vi "FFT Simulation test.vi"   [LabVIEW 2014]
uses:
  <vilib>/Platform/TimedLoop/XDataNode/timing_clust.ctl
  <vilib>/Platform/TimedLoop/XDataNode/nitl_modes.ctl
  <vilib>/Platform/TimedLoop/XDataNode/wakeup.ctl
  <vilib>/rvi/Analysis/measure/FFT/simModelSupport/niFPGA FFT Streaming Sim Properties.ctl
  <vilib>/rvi/Analysis/measure/FFT/simModelSupport/niFPGA FFT Sim Stream Group Properties.ctl
  <vilib>/rvi/Analysis/measure/FFT/simModelSupport/niFPGA FFT Sim Types.ctl
  <vilib>/rvi/Analysis/measure/FFT/simModelSupport/niFpgaFFTSimArithmeticProperties.ctl
  <vilib>/rvi/Analysis/measure/FFT/simModelSupport/niFpgaFFTSimDfxp.ctl
  <vilib>/fxp/LVFixedPointQuantizationPolicyTypeDef.ctl
  <vilib>/rvi/Analysis/measure/FFT/XNode/niFpgaFFTButterflyDelays.ctl
  <vilib>/rvi/Emulation/niFpgaSctlEmulationGetInTimedLoop.vi
  <vilib>/rvi/Emulation/niFpgaEmulationReportErrorSimple.vi
  <vilib>/rvi/Emulation/niFpgaGetClockAttributes.vi
  <vilib>/rvi/Emulation/niFpgaCriticalErrorInLSC.vi
  <vilib>/rvi/Memory/Memory_Emulation/nirvimemoryFastEmulation.vi
  <vilib>/rvi/Memory/Memory_Emulation/nirvimemoryEmulation.vi
  <vilib>/rvi/Emulation/niFpgaEmulationIsFPGAContextNoSignature.vi
  <vilib>/rvi/DataTransferAndStorage/Container/Common/niFpgaContainerGetUniqueNameForEmu.vi
  <vilib>/rvi/Emulation/niFpgaProcessEmulError.vi
  <vilib>/rvi/errors/nirviReportUnexpectedCaseInternalError (U32).vi
  <vilib>/rvi/interface/RandomDataEmulation/niFpgaRandomDataHandleErrors.vi
  <vilib>/rvi/errors/niFpgaSetErrorForExecOnDevCompSimple.vi
  <vilib>/rvi/eio/common/nirviEmuReportErrorAndStop.vi
  <vilib>/rvi/FIFO/Fifo_Resource/nirvififoEmulationSetSize.vi
  <vilib>/rvi/FIFO/Fifo_Resource/nirviFifoEmulationQueueMgr.vi
  <instcachedir>/0/nirviFifoEmulationQueueMgr_E5CAEC123FF24DC58D834DCA3CDAA9B5.lvgen/nirviFifoEmulationQueueMgr_E5CAEC123FF24DC58D834DCA3CDAA9B5_010.vi
  <vilib>/rvi/FIFO/Fifo_Resource/nirvififoEmulationDetermineInputValidOut.vi
  <vilib>/rvi/FIFO/Fifo_Resource/nirvififoEmulationCreateLock.vi
  <vilib>/rvi/FIFO/Fifo_Resource/nirvififoEmulationObtainLock.vi
  <vilib>/rvi/FIFO/Fifo_Resource/nirvififoEmulationReleaseLock.vi
  <vilib>/rvi/occurrence/nirviWaitOnOccurrenceBase.vi
  <vilib>/rvi/errors/nirviReportUnexpectedCaseInternalError.vi
  <vilib>/rvi/Analysis/measure/FFT/simModelSupport/niFpgaFFTSimModelStreamingCore.vi
  <vilib>/Platform/TimedLoop/XDataNode/XDataNode.xnode
  <vilib>/rvi/DataTransferAndStorage/Container/XNode/niFpgaContainer.xnode
  <vilib>/rvi/interface/RandomDataEmulation/nirviRandomDataFpgaReadWriteTemplate.vi
  <vilib>/rvi/FIFO/Fifo_Resource/nirvififoEmulationWrite.vi
  <vilib>/rvi/FIFO/Fifo_Resource/nirvififoEmulationRead.vi
  <vilib>/rvi/Analysis/measure/FFT/XNode/niFpgaFFT.xnode
  <vilib>/Platform/TimedLoop/XDataNode/XDNodeRunTimeDep.lvlib
types:
  T1 = typedef "XDNodeRunTimeDep.lvlib/timing_clust.ctl" = cluster{"Expected End [f-1]":u64, "Actual End [f-1]":u64, "Finished Late? [f-1]":bool, "Expected End [i-1]":u64, "Actual End [i-1]":u64, "Finished Late? [i-1]":bool, "Expected Start [i]":u64, "Actual Start [i]":u64, "Expected Start [f]":u64, "Actual Start [f]":u64, "Source Name":string, "Structure Name":string, "Period":i64, "Deadline":i64, "Offset":i64, "Start":i64, "Priority":i32, "Timeout":i32, "Mode":T2, "Wakeup Reason":T3, "Error":errorcluster, "Source Type":string, "Secondary Source Type":string, "Global End Time":u64, "Global Start Time":u64, "Frame Duration":u64, "Iteration Duration":u64, "Assigned CPU":i32, "I/O Scan Engine Mode":u32}
  T2 = typedef "XDNodeRunTimeDep.lvlib/nitl_modes.ctl" = enum32{"No Change", "Process missed periods, maintain original phase", "Discard missed periods, maintain original phase", "Process missed periods, ignore original phase", "Discard missed periods, ignore original phase"}
  T3 = typedef "XDNodeRunTimeDep.lvlib/wakeup.ctl" = enum32{"Normal", "Aborted", "Asynchronous wakeup", "Timing source error", "Timed loop error", "Timeout"}
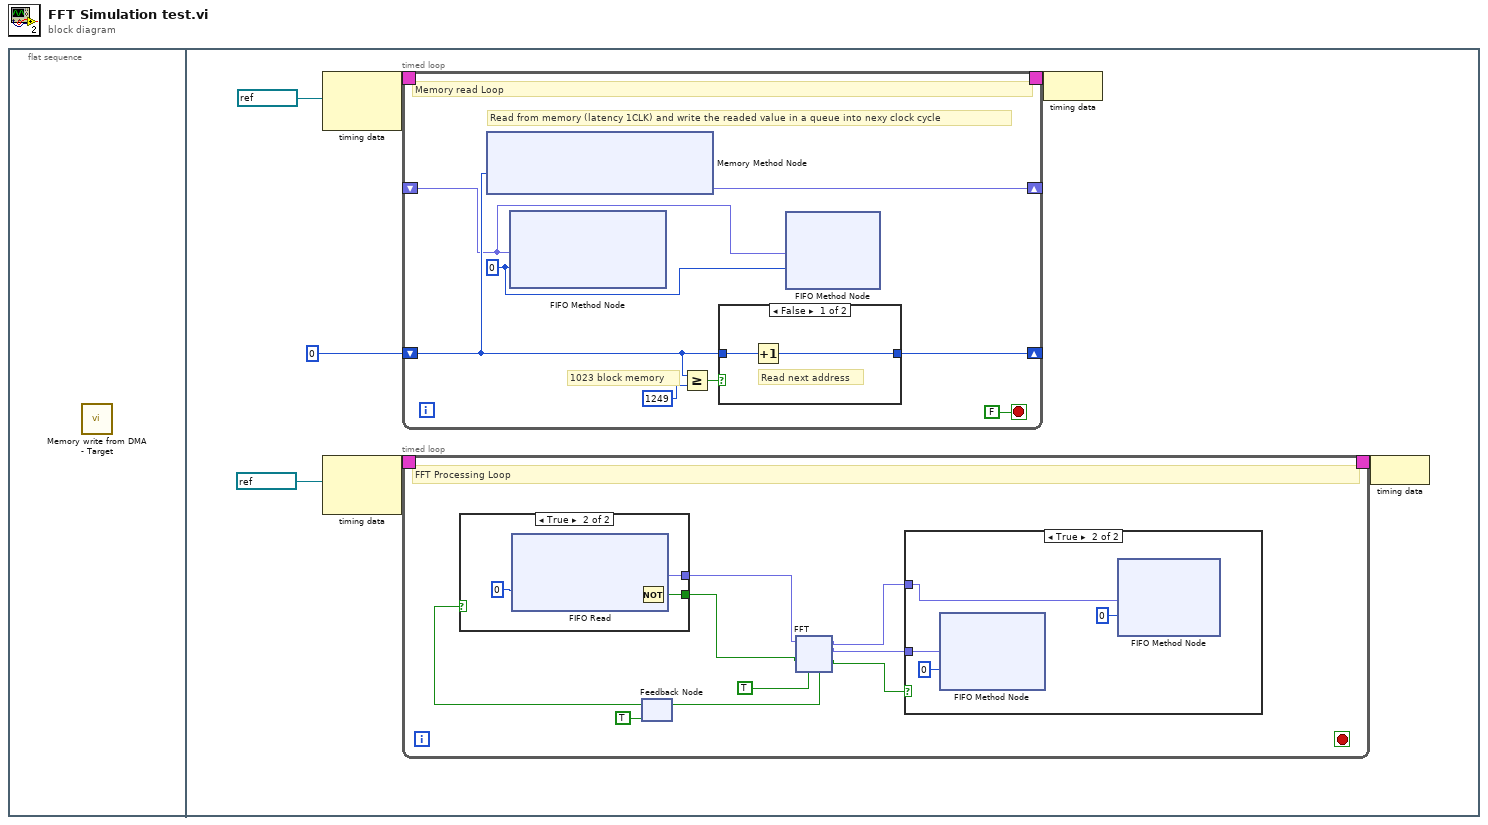
[diagram p0: block diagram]
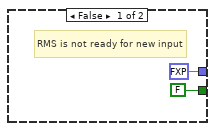
[diagram p3: hidden frame]
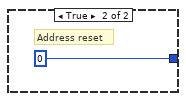
[diagram p4: hidden frame]
diagram:
  n1 = flat-sequence {
    frame #0 {
      n2 = call "Memory write from DMA - Target.vi"() -> ()  [unwired: 12 in]
    }
    frame #1 {
      n3 = node-c288(refnum<k21> "50MHz" ("Source Name")) -> (w7:T1)  [unwired: 1 in]
      n4 = node-c288(refnum<k21> "50MHz" ("Source Name")) -> (w5:T1)  [unwired: 1 in]
      n5 = timed-loop {
        timing: w7 -> [_]
        timing-out: [_] -> w6
        shift-right: [w66] -> _
        shift-left: _ -> [w60]
        shift-right: [w63] -> _
        shift-left: u32 0 -> [w61]
        stop <- FALSE stop-if-true
        w59 = 0 ("Timeout")
        # "1023 block memory"
        # "Read from memory (latency 1CLK) and write the readed value in a queue into nexy clock cycle"
        # "Memory read Loop"
        n6 = xnode ("Memory Method Node")("Address"=w61) -> ("Data"=w66:fxp<+/-,12,12>)  [unwired: 1 in, 1 out]
        n7 = xnode ("FIFO Method Node")("Element"=w60, "Timeout"=w59) -> ()  [unwired: 1 in, 2 out]
        n8 = Greater Or Equal?(x=w61, y=u32 1249) -> (x >= y?=w64:bool)
        n9 = case shown="False" w64 {
          tunnel: w61 -> [w68 _]
          tunnel: [w67 u32 0] -> w63
          frame False {
            # "Read next address"
            n10 = Increment(x=w68) -> (x+1=w67:u32)
          }
          frame True {
            # "Address reset"
          }
        }
        n11 = xnode ("FIFO Method Node")("Element"=w60, "Timeout"=w59) -> ()  [unwired: 1 in, 2 out]
      }
      n12 = timed-loop {
        timing: w5 -> [_]
        timing-out: [_] -> w4
        stop <- _ stop-if-true
        # "FFT Processing Loop"
        n13 = feedback #1(TRUE ("ready for input")) -> (w16:bool)
        n14 = case shown="True" w16 {
          tunnel: [FALSE w52] -> w8
          tunnel: [fxp<+/-,12,12> 0.0 ("Element") w49] -> w14
          frame False {
            # "RMS is not ready for new input"
          }
          frame True {
            n15 = xnode ("FIFO Read")("Timeout"=0) -> ("Element"=w49:fxp<+/-,12,12>, "Timed Out?"=w51:bool)  [unwired: 1 in, 1 out]
            n16 = Not(x=w51) -> (.not. x?=w52:bool)
          }
        }
        n17 = xnode "FFT"("real data in"=w14, "input valid"=w8, "ready for output"=TRUE) -> ("ready for input"=w10:bool, "real data out"=w13:fxp<+/-,22,22>, "imaginary data out"=w12:fxp<+/-,22,22>, "output valid"=w11:bool)  [unwired: 2 in, 1 out]
        n18 = feedback-in #1(w10) -> ()
        n19 = case shown="True" w11 {
          tunnel: w13 -> [_ w45]
          tunnel: w12 -> [_ w46]
          frame False {
          }
          frame True {
            n20 = xnode ("FIFO Method Node")("Element"=w46, "Timeout"=0) -> ()  [unwired: 1 in, 2 out]
            n21 = xnode ("FIFO Method Node")("Element"=w45, "Timeout"=0) -> ()  [unwired: 1 in, 2 out]
          }
        }
      }
      n22 = node-c288(w6) -> ()
      n23 = node-c288(w4) -> ()
    }
  }
